vi "Refresh Feed (By Name).vi"(8 "error in":errorcluster, 11 "feed name in":string) -> (0 "error out":errorcluster, 3 "feed name out":string)   [LabVIEW 2014, in "NIPM_API.lvlib"]
doc: "Refreshes NI Package Manager with data from the specified feed. \n\nFeed name - This input must refer to a registered feed. This input cannot be an empty string.\nNote: Feed names are case-sensitive."
uses:
  NIPM_API.lvlib
panel:
  out "command line standard output":string
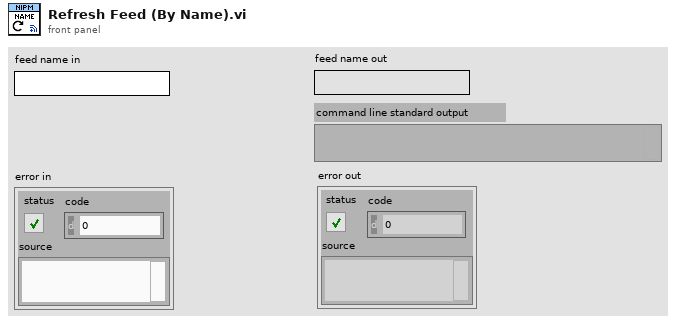
[diagram p1: front panel]
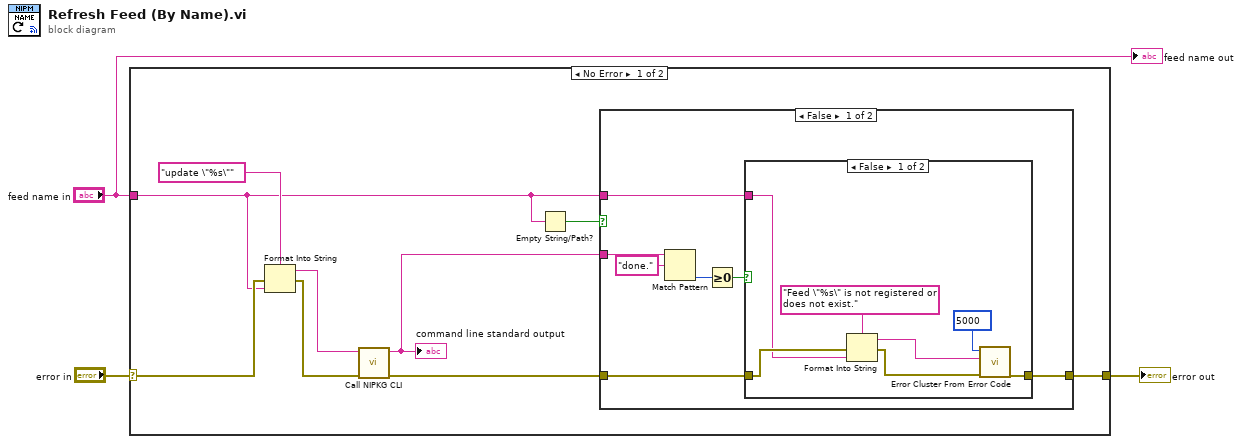
[diagram p0: block diagram]
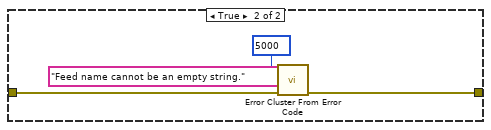
[diagram p3: hidden frame]
diagram:
  n1 = case shown="No Error" "error in" {
    selector: "error in" -> [w10 w32]
    tunnel: [w5 w32] -> w2
    tunnel: "feed name in" -> [w4 _]
    frame No Error {
      n2 = Format Into String(format string="update \"%s\"", error in=w10, w4) -> (resulting string=w11:string, error out=w9:errorcluster)  [unwired: 1 in]
      n3 = call "Call NIPKG CLI.vi"("error in (no error)"=w9, "command"=w11) -> ("error out"=w7:errorcluster, "command line standard output"=w6:string)  [unwired: 8 in]
      "command line standard output" <- w6
      n4 = Empty String/Path?(string/path=w4) -> (empty?=w8:bool)
      n5 = case shown="False" w8 {
        tunnel: w7 -> [w15 w30]
        tunnel: [w14 w29] -> w5
        tunnel: w6 -> [w18 _]
        tunnel: w4 -> [w13 _]
        frame False {
          n6 = Match Pattern(string=w18, regular expression="done." ("search string")) -> (offset past match=w17:i32)  [unwired: 1 in, 3 out]
          n7 = Greater Or Equal To 0?(x=w17) -> (x >= 0?=w16:bool)
          n8 = case shown="False" w16 {
            tunnel: w15 -> [w22 w27]
            tunnel: [w21 w27] -> w14
            tunnel: w13 -> [w20 _]
            frame False {
              n9 = Format Into String(format string="Feed \"%s\" is not registered or does not exist.", error in=w22, w20) -> (resulting string=w23:string, error out=w24:errorcluster)  [unwired: 1 in]
              n10 = call <vilib>:"Error Cluster From Error Code.vi"("error in (no error)"=w24, "error message (\"\")"=w23, "error code (0)"=5000) -> ("error out"=w21:errorcluster)  [unwired: 6 in]
            }
            frame True {
              # "Resync occurred successfully."
            }
          }
        }
        frame True {
          n11 = call <vilib>:"Error Cluster From Error Code.vi"("error in (no error)"=w30, "error message (\"\")"="Feed name cannot be an empty string." ("error message (\"\")"), "error code (0)"=5000) -> ("error out"=w29:errorcluster)  [unwired: 6 in]
        }
      }
    }
    frame Error {
    }
  }
  "error out" <- w2
  "feed name out" <- "feed name in"
